vi "Controller Apply Configuration from GUI.vi"(7 "Sync Objects":T3, 8 "error in (no error)":errorcluster, 10 "Configuration Data (GUI to Controller)":T2) -> (0 "error out":errorcluster, 2 "Configuration Change Acknowledge (Controller to GUI)":T1)   [LabVIEW 2011, in "Controller VIs.lvlib"]
uses:
  Controller VIs.lvlib
  Types Definitions/Type Synchronization Objects.ctl
  Types Definitions/Type Blocking Synchronization Objects.ctl
  Types Definitions/Type FA Request Parameters.ctl
  Types Definitions/Type BPM and PS select cluster.ctl
  Types Definitions/Type FA File Parameters.ctl
  Types Definitions/Type Monitoring Data.ctl
  Types Definitions/Type Diagnostics Data.ctl
  Types Definitions/Type CPU Loads Array.ctl
  Types Definitions/Type CPU Loads.ctl
  Types Definitions/Type Non-blocking Synchronization Objects.ctl
  Types Definitions/Type FOFB Variables.ctl
  Types Definitions/Type Actuation State.ctl
  Types Definitions/Type Configuration Data (GUI to Controller).ctl
  Types Definitions/Type Configuration Change Acknowledge (Controller to GUI).ctl
  Types Definitions/Type PID Parameters.ctl
  Types Definitions/Type FOFB Configuration.ctl
  Types Definitions/Type FOFB Parameters.ctl
  Types Definitions/Type Network Configuration.ctl
  Types Definitions/Type FA Configuration.ctl
  Types Definitions/Type Response Matrix Measurement Configuration.ctl
  Types Definitions/Type Correction Algorithm Configuration.ctl
  Types Definitions/Type Acquisition Network Configuration.ctl
  Types Definitions/Type Actuation Network Configuration.ctl
  Type Definitions.lvlib
  XML VIs.lvlib
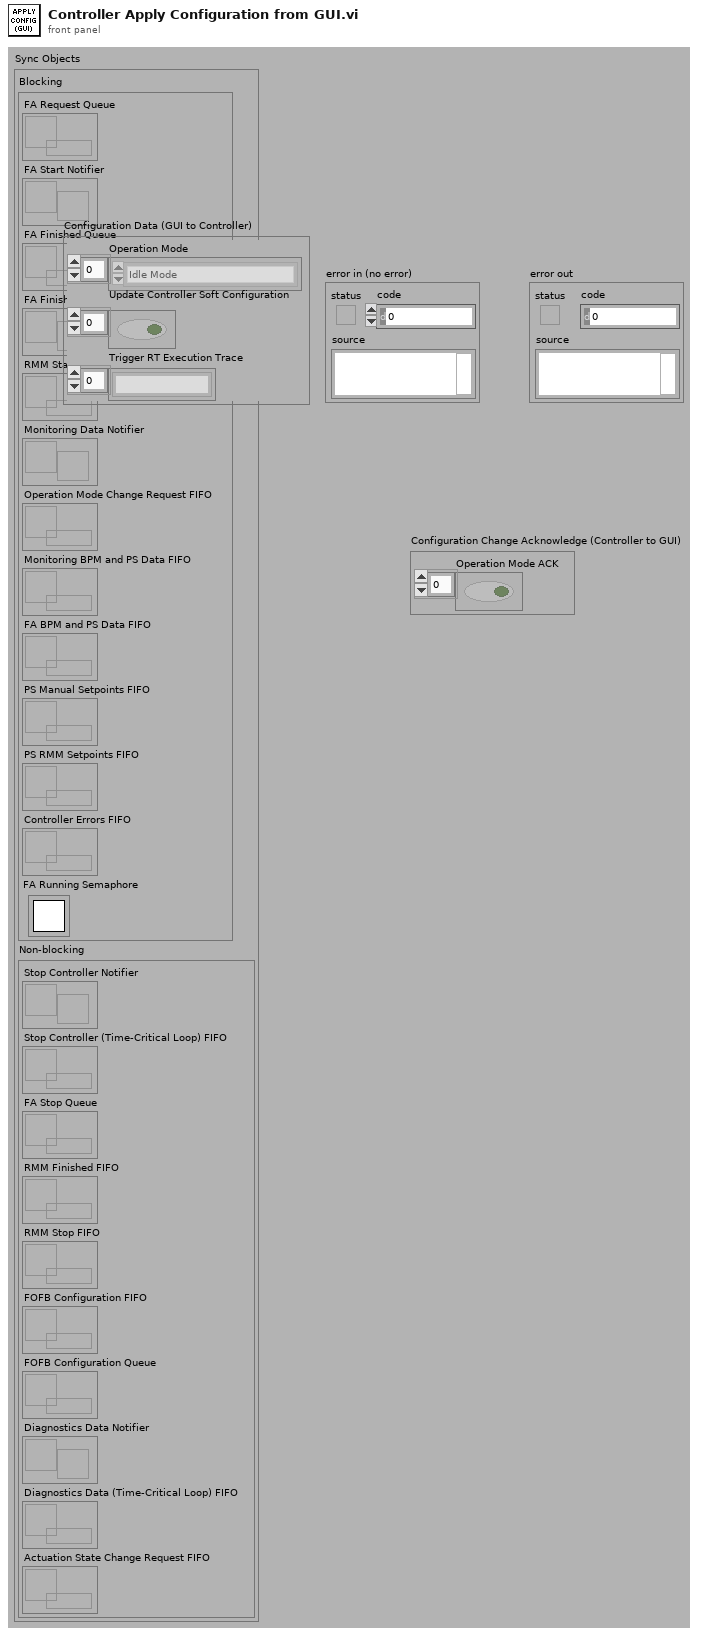
[diagram p1: front panel]
types:
  T1 = typedef "Type Definitions.lvlib/Type Configuration Change Acknowledge (Controller to GUI).ctl" = cluster{"Operation Mode ACK":bool[]}
  T2 = typedef "Type Definitions.lvlib/Type Configuration Data (GUI to Controller).ctl" = cluster{"Operation Mode":enum16{"Idle Mode", "Error Mode", "Manual Mode", "FOFB Mode", "RMM Mode"}[], "Update Controller Soft Configuration":bool[], "Trigger RT Execution Trace":string[]}
  T3 = typedef "Type Definitions.lvlib/Type Synchronization Objects.ctl" = cluster{"Blocking":T4, "Non-blocking":T6}
  T4 = typedef "Type Definitions.lvlib/Type Blocking Synchronization Objects.ctl" = cluster{"FA Request Queue":refnum<queue>, "FA Start Notifier":refnum<notifier>, "FA Finished Queue":refnum<queue>, "FA Finished Broadcast Notifier":refnum<notifier>, "RMM Start FIFO":refnum<k33>, "Monitoring Data Notifier":refnum<notifier>, "Operation Mode Change Request FIFO":refnum<k33>, "Monitoring BPM and PS Data FIFO":refnum<k33>, "FA BPM and PS Data FIFO":refnum<k33>, "PS Manual Setpoints FIFO":refnum<k33>, "PS RMM Setpoints FIFO":refnum<k33>, "Controller Errors FIFO":refnum<k33>, "FA Running Semaphore":T5}
  T5 = typedef "Semaphore RefNum" = refnum<k1>
  T6 = typedef "Type Definitions.lvlib/Type Non-blocking Synchronization Objects.ctl" = cluster{"Stop Controller Notifier":refnum<notifier>, "Stop Controller (Time-Critical Loop) FIFO":refnum<k33>, "FA Stop Queue":refnum<queue>, "RMM Finished FIFO":refnum<k33>, "RMM Stop FIFO":refnum<k33>, "FOFB Configuration FIFO":refnum<k33>, "FOFB Configuration Queue":refnum<queue>, "Diagnostics Data Notifier":refnum<notifier>, "Diagnostics Data (Time-Critical Loop) FIFO":refnum<k33>, "Actuation State Change Request FIFO":refnum<k33>}
  T7 = typedef "Type Definitions.lvlib/Type PID Parameters.ctl" = cluster{"Kc":fxp<+/-,16,8>, "Ti":fxp<+/-,16,8>, "Td":fxp<+/-,16,8>}
  T8 = cluster{"Number of Acquisition Chassis":i32, "Number of Actuation Chassis":i32, "Number of BPM Readings":i32, "BPM Reading Names":string[], "Selected BPM Readings":u32[], "Number of Correctors":i32, "Corrector Names":string[], "Selected Correctors":u32[], "Reference Orbit":dbl[], "Response Matrix":dbl[][], "Correction Matrix":dbl[][], "Acquisition Chassis Names":string[], "Actuation Chassis Names":string[], "Acquisition Variables":cluster{"Variable Name":string, "Chassis Name":string}[], "Actuation Variables":cluster{"Variable Name":string, "Chassis Name":string}[], "PS Matrix Mapping":cluster{u32[]}[], "Inverse PS Matrix Mapping":u32[][], "Response Matrix Beam Energy (MeV)":dbl, "PID Parameters":T7[], "BPM Planes":enum8{"H", "V"}[], "Corrector Planes":enum8{"H", "V"}[], "RMM Step Factor":dbl[]}
  T9 = enum16{"Idle Mode", "Error Mode", "Manual Mode", "FOFB Mode", "RMM Mode"}[]
  T10 = enum16{"Idle Mode", "Error Mode", "Manual Mode", "FOFB Mode", "RMM Mode"}
  T11 = typedef "Type Definitions.lvlib/Type FOFB Configuration.ctl" = cluster{"FOFB Parameters":T12, "Number of Acquisition Chassis":i32, "Number of Actuation Chassis":i32, "Number of BPM Readings":i32, "BPM Reading Names":string[], "Selected BPM Readings":u32[], "Number of Correctors":i32, "Corrector Names":string[], "Selected Correctors":u32[], "Reference Orbit":dbl[], "Response Matrix":dbl[][], "Correction Matrix":dbl[][], "Acquisition Chassis Names":string[], "Actuation Chassis Names":string[], "Acquisition Variables":cluster{"Variable Name":string, "Chassis Name":string}[], "Actuation Variables":cluster{"Variable Name":string, "Chassis Name":string}[], "PS Matrix Mapping":cluster{u32[]}[], "Inverse PS Matrix Mapping":u32[][], "Response Matrix Beam Energy (MeV)":dbl, "PID Parameters":T7[], "BPM Planes":enum8{"H", "V"}[], "Corrector Planes":enum8{"H", "V"}[], "RMM Step Factor":dbl[]}
  T12 = typedef "Type Definitions.lvlib/Type FOFB Parameters.ctl" = cluster{"Network":T13, "Fast Acquisition":T14, "Response Matrix Measurement":T15, "Correction Algorithm":T16, "Acquisition Network":T17, "Actuation Network":T18}
  T13 = typedef "Type Definitions.lvlib/Type Network Configuration.ctl" = cluster{"FOFB Controller IP":string, "LNLS Control Network IP":string, "LNLS Control Network Power Supplies TCP Port":u16, "LNLS Control Network FOFB Configuration TCP Port":u16, "Data Server TCP Port":u16, "Monitoring Data TCP Port":u16, "Configuration GUI TCP Port":u16, "TCP Listening Timeout":i32}
  T14 = typedef "Type Definitions.lvlib/Type FA Configuration.ctl" = cluster{"Acquisition Period":u32, "Data Buffer Size":u32}
  T15 = typedef "Type Definitions.lvlib/Type Response Matrix Measurement Configuration.ctl" = cluster{"Step Amplitude":dbl, "Time Between Steps":u32, "Step Duration":u32, "Number of Averages":u32}
  T16 = typedef "Type Definitions.lvlib/Type Correction Algorithm Configuration.ctl" = cluster{"Correction Period":u32, "Reference Orbit Path":path, "Response Matrix Path":path, "Correction Matrix Path":path, "Horizontal Correction Factor":dbl, "Vertical Correction Factor":dbl, "Beam Current FOFB Threshold":dbl, "Decouple H-V":bool}
  T17 = typedef "Type Definitions.lvlib/Type Acquisition Network Configuration.ctl" = cluster{"Chassis Name":string, "Variables":cluster{"Variable Name":string, "Matrix Order":u32, "Location":dbl, "Plane":enum8{"H", "V"}, "On Correction":bool}[]}[]
  T18 = typedef "Type Definitions.lvlib/Type Actuation Network Configuration.ctl" = cluster{"Chassis Name":string, "Variables":cluster{"Variable Name":string, "Matrix Order":u32, "RMM Step Factor":dbl, "Plane":enum8{"H", "V"}, "On Correction":bool, "Kc":dbl, "Ti":dbl, "Td":dbl}[]}[]
  T19 = typedef "Type Definitions.lvlib/Type FOFB Variables.ctl" = cluster{"Correction Period":u32, "Reference Orbit":dbl[], "Response Matrix":dbl[][], "Correction Matrix":dbl[][], "Decouple H-V":bool, "Horizontal Correction Factor":dbl, "Vertical Correction Factor":dbl, "Selected BPM Readings":u32[], "Selected Correctors":u32[], "BPM Planes":enum8{"H", "V"}[], "Corrector Planes":enum8{"H", "V"}[], "Beam Current FOFB Threshold":dbl, "Response Matrix Beam Energy (MeV)":dbl}
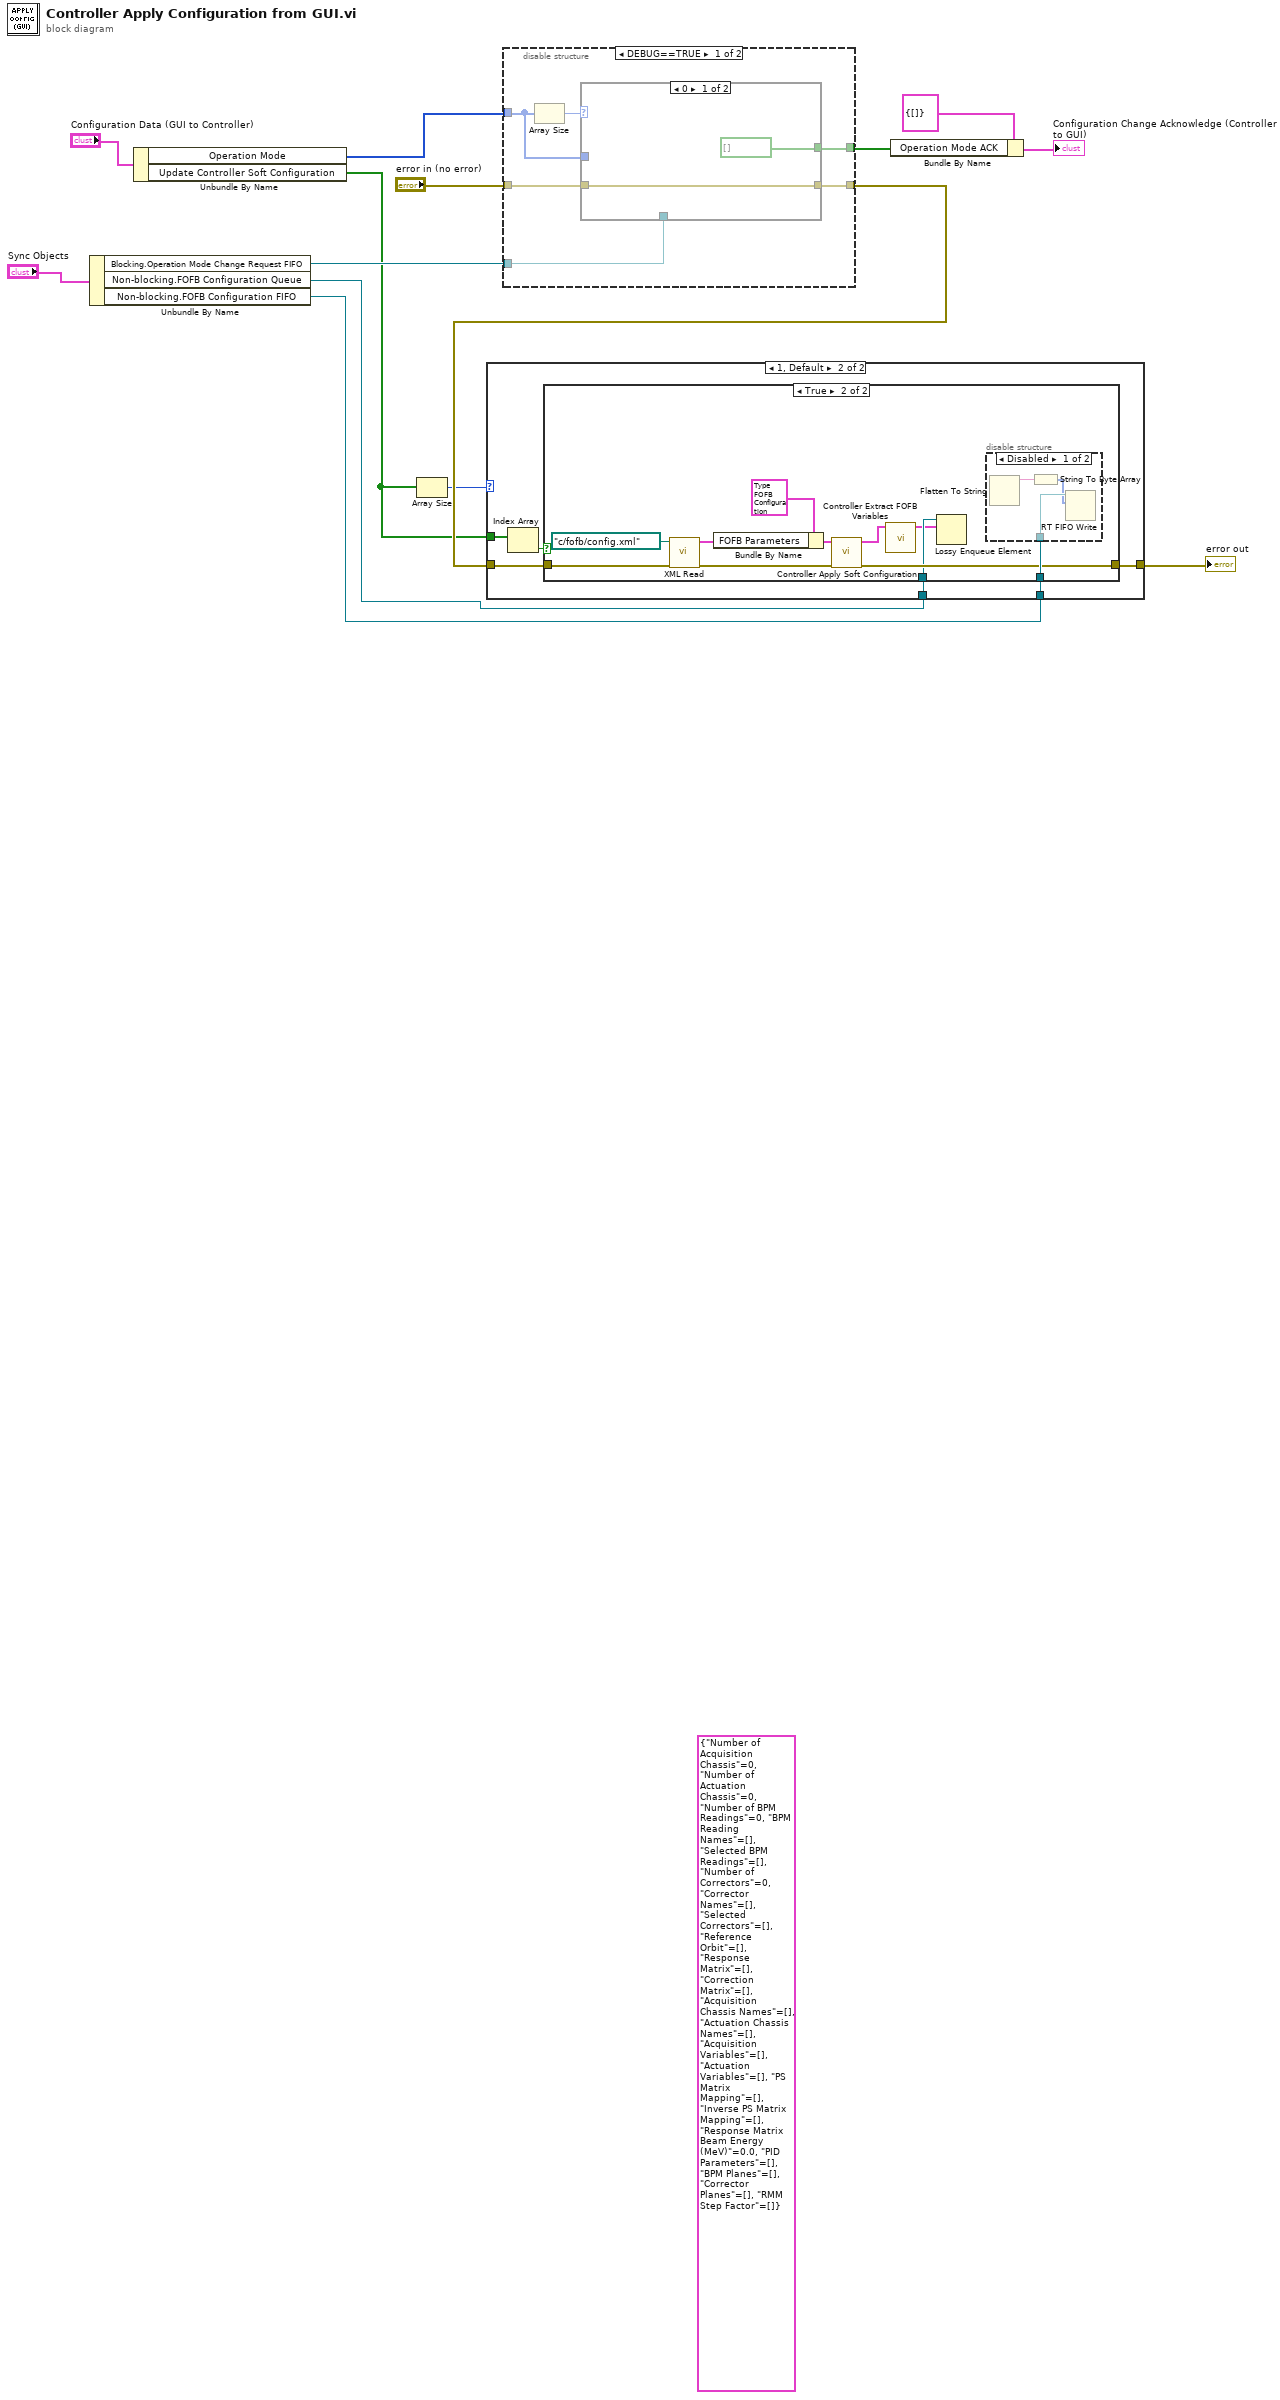
[diagram p0: block diagram]
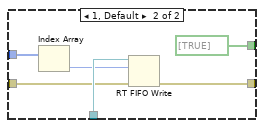
[diagram p2: hidden frame]
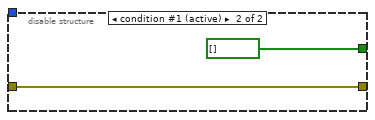
[diagram p3: hidden frame]
diagram:
  (unwired) T8 {"Number of Acquisition Chassis"=0, "Number of Actuation Chassis"=0, "Number of BPM Readings"=0, "BPM Reading Names"=[], "Selected BPM Readings"=[], "Number of Correctors"=0, "Corrector Names"=[], "Selected Correctors"=[], "Reference Orbit"=[], "Response Matrix"=[], "Correction Matrix"=[], "Acquisition Chassis Names"=[], "Actuation Chassis Names"=[], "Acquisition Variables"=[], "Actuation Variables"=[], "PS Matrix Mapping"=[], "Inverse PS Matrix Mapping"=[], "Response Matrix Beam Energy (MeV)"=0.0, "PID Parameters"=[], "BPM Planes"=[], "Corrector Planes"=[], "RMM Step Factor"=[]} ("cluster")
  n1 = Unbundle By Name("Sync Objects") -> ("Blocking.Operation Mode Change Request FIFO"=w13:refnum<k33>, "Non-blocking.FOFB Configuration Queue"=w1:refnum<queue>, "Non-blocking.FOFB Configuration FIFO"=w2:refnum<k33>)
  n2 = Unbundle By Name("Configuration Data (GUI to Controller)") -> ("Operation Mode"=w11:T9, "Update Controller Soft Configuration"=w3:bool[])
  n3 = Array Size(array=w3) -> (size(s)=w4:i32)
  n4 = disable-structure shown="DEBUG==TRUE" {
    disable-tunnel: w13 -> [w20 _]
    disable-tunnel: "error in (no error)" -> [w19 w30]
    disable-tunnel: w11 -> [w18 _]
    disable-tunnel: [w16 bool[] [] ("Operation Mode ACK")] -> w7
    disable-tunnel: [w15 w30] -> w6
    frame condition #0 {
      n5 = Array Size(array=w18) -> (size(s)=w17:i32)
      n6 = case shown="0" w17 {
        tunnel: w18 -> [_ w28]
        tunnel: w20 -> [_ w27]
        tunnel: w19 -> [w22 w26]
        tunnel: [w22 w25] -> w15
        tunnel: [bool[] [] ("Operation Mode ACK") bool[] [TRUE] ("Operation Mode ACK")] -> w16
        frame 0 {
        }
        frame 1, Default {
          n7 = Index Array(array=w28) -> (element=w23:T10)  [unwired: 1 in]
          n8 = RT FIFO Write(0:w27, 1:w23, 3:w26) -> (11:w25:errorcluster)  [unwired: 2 in, 3 out]
        }
      }
    }
    frame condition #1 (active) {
    }
  }
  n9 = case shown="1, Default" w4 {
    tunnel: w3 -> [_ w37]
    tunnel: w6 -> [w31 w35]
    tunnel: [w31 w34] -> w5
    tunnel: w2 -> [_ w33]
    tunnel: w1 -> [_ w32]
    frame 0 {
    }
    frame 1, Default {
      n10 = Index Array(array=w37) -> (element=w36:bool)  [unwired: 1 in]
      n11 = case shown="True" w36 {
        tunnel: w35 -> [w38 w45]
        tunnel: [w38 w43] -> w34
        tunnel: w33 -> [_ w44]
        tunnel: w32 -> [_ w41]
        frame False {
        }
        frame True {
          n12 = call "XML Read.vi"("error in"=w45, "XML File Path In"=path "c:/fofb/config.xml" ("Configuration File Path")) -> ("error out"=w48:errorcluster, "FOFB Parameters"=w46:T12)  [unwired: 8 in]
          n13 = Bundle By Name(cluster=T11 {"FOFB Parameters"={"Network"={"FOFB Controller IP"="", "LNLS Control Network IP"="", "LNLS Control Network Power Supplies TCP Port"=0, "LNLS Control Network FOFB Configuration TCP Port"=0, "Data Server TCP Port"=0, "Monitoring Data TCP Port"=0, "Configuration GUI TCP Port"=0, "TCP Listening Timeout"=0}, "Fast Acquisition"={"Acquisition Period"=0, "Data Buffer Size"=0}, "Response Matrix Measurement"={"Step Amplitude"=0.0, "Time Between Steps"=0, "Step Duration"=0, "Number of Averages"=0}, "Correction Algorithm"={"Correction Period"=0, "Reference Orbit Path"=path "", "Response Matrix Path"=path "", "Correction Matrix Path"=path "", "Horizontal Correction Factor"=0.0, "Vertical Correction Factor"=0.0, "Beam Current FOFB Threshold"=0.0, "Decouple H-V"=FALSE}, "Acquisition Network"=[], "Actuation Network"=[]}, "Number of Acquisition Chassis"=0, "Number of Actuation Chassis"=0, "Number of BPM Readings"=0, "BPM Reading Names"=[], "Selected BPM Readings"=[], "Number of Correctors"=0, "Corrector Names"=[], "Selected Correctors"=[], "Reference Orbit"=[], "Response Matrix"=[], "Correction Matrix"=[], "Acquisition Chassis Names"=[], "Actuation Chassis Names"=[], "Acquisition Variables"=[], "Actuation Variables"=[], "PS Matrix Mapping"=[], "Inverse PS Matrix Mapping"=[], "Response Matrix Beam Energy (MeV)"=0.0, "PID Parameters"=[], "BPM Planes"=[], "Corrector Planes"=[], "RMM Step Factor"=[]}, "FOFB Parameters"=w46) -> (w47:T11)
          n14 = call "Controller Apply Soft Configuration.vi"("error in (no error)"=w48, "FOFB Configuration"=w47) -> ("error out"=w43:errorcluster, "FOFB Configuration"=w42:T11)  [unwired: 8 in]
          n15 = call "Controller Extract FOFB Variables.vi"("FOFB Configuration"=w42) -> ("FOFB Variables"=w39:T19)  [unwired: 9 in, 1 out]
          n16 = Lossy Enqueue Element(queue=w41, element=w39) -> ()  [unwired: 1 in, 4 out]
          n17 = disable-structure shown="Disabled" {
            disable-tunnel: w44 -> [w52 _]
            frame Disabled {
              n18 = Flatten To String() -> (data string=w51:string)  [unwired: 4 in, 2 out]
              n19 = String To Byte Array(string=w51) -> (unsigned byte array=w50:u8[])
              n20 = RT FIFO Write(0:w52, 1:w50) -> ()  [unwired: 3 in, 4 out]
            }
            frame Enabled {
            }
          }
        }
      }
    }
  }
  "error out" <- w5
  n21 = Bundle By Name(cluster=T1 {"Operation Mode ACK"=[]} ("Configuration Change Acknowledge (Controller to GUI)"), "Operation Mode ACK"=w7) -> (→"Configuration Change Acknowledge (Controller to GUI)":T1)
